vi "Get.vi"(8 "error in (no error)":errorcluster, 10 "valve in":T2=7 items=["Valve 1"=1, "Valve 2"=2, "Valve 3"=3, "Valve 4"=4, "Valve 5"=5, "Valve 6"=6, "Valve 7"=7], 11 "INL Valve Controller in":refnum<class "INL Valve Controller.lvclass">) -> (0 "error out":errorcluster, 1 "status out":T1 items=["Closed", "Open"], 2 "valve out":T2=7 items=["Valve 1"=1, "Valve 2"=2, "Valve 3"=3, "Valve 4"=4, "Valve 5"=5, "Valve 6"=6, "Valve 7"=7], 3 "INL Valve Controller out":refnum<class "INL Valve Controller.lvclass">)   [LabVIEW 2011, in "INL Valve Controller.lvclass"]
uses:
  INL Valve Controller.lvclass
  Valve Controller/Valves.ctl
  Valve Controller/Status.ctl
  INL Valve Controller.lvclass/INL Valve Controller.ctl
  Valve Controller/Valve Controller.lvclass
panel:
  out "read buffer":string
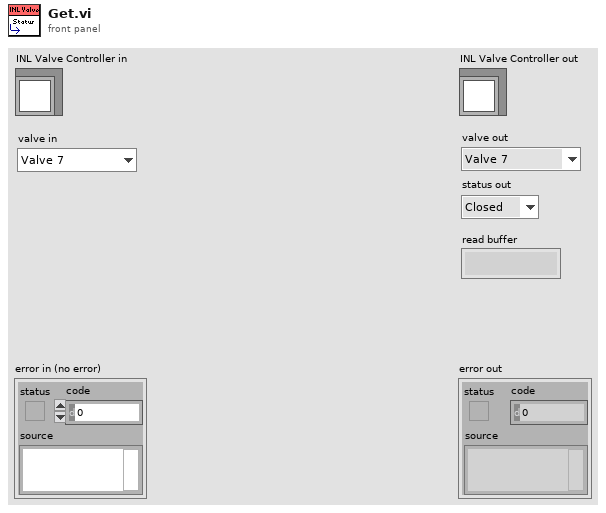
[diagram p1: front panel]
types:
  T1 = typedef "Valve Controller.lvclass/Status.ctl" = u16
  T2 = typedef "Valve Controller.lvclass/Valves.ctl" = u16
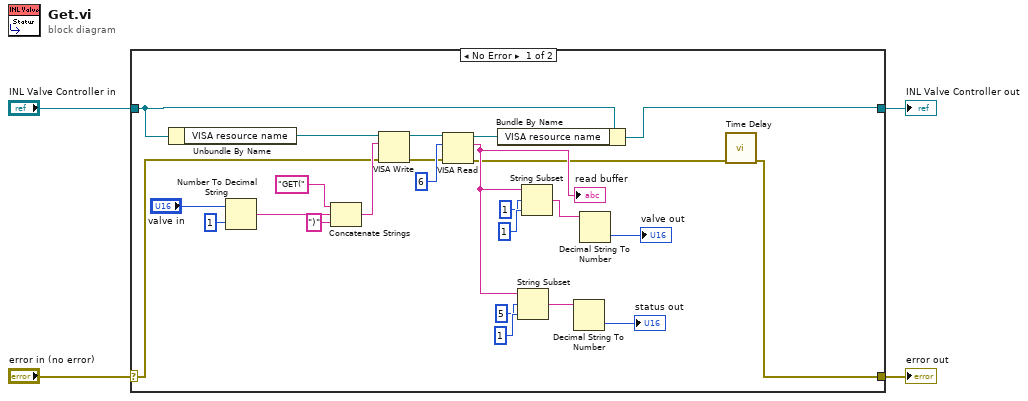
[diagram p0: block diagram]
diagram:
  n1 = case shown="No Error" "error in (no error)" {
    selector: "error in (no error)" -> [w6 w31]
    tunnel: [w5 w31] -> w3
    tunnel: [w7 w30] -> w1
    tunnel: "INL Valve Controller in" -> [w8 w30]
    frame No Error {
      n2 = Unbundle By Name(w8) -> ("VISA resource name"=w9:refnum<visa-resource-name>)
      n3 = Number To Decimal String(number="valve in", width (-)=i16 1) -> (decimal integer string=w28:string)
      n4 = Concatenate Strings("GET(", w28, ")" ("string")) -> (w26:string)
      n5 = VISA Write(VISA resource name=w9, write buffer=w26, error in (no error)=w6) -> (VISA resource name out=w18:refnum<visa-resource-name>, error out=w15:errorcluster)  [unwired: 1 out]
      n6 = VISA Read(VISA resource name=w18, byte count=u32 6, error in (no error)=w15) -> (VISA resource name out=w17:refnum<visa-resource-name>, read buffer=w14:string, error out=w10:errorcluster)  [unwired: 1 out]
      "read buffer" <- w14
      n7 = Bundle By Name(cluster=w8, "VISA resource name"=w17) -> (w7:refnum<class "INL Valve Controller.lvclass">)
      n8 = String Subset(string=w14, offset (0)=5, length (rest)=1 ("length (rest)")) -> (substring=w19:string)
      n9 = String Subset(string=w14, offset (0)=1, length (rest)=1 ("length (rest)")) -> (substring=w22:string)
      n10 = Decimal String To Number(string=w19) -> (number=→"status out":i32)  [unwired: 2 in, 1 out]
      n11 = Decimal String To Number(string=w22) -> (number=→"valve out":i32)  [unwired: 2 in, 1 out]
      n12 = call "Time Delay"("error in (no error)"=w10) -> ("error out"=w5:errorcluster)  [unwired: 10 in]
    }
    frame Error {
    }
  }
  "error out" <- w3
  "INL Valve Controller out" <- w1
